vi "PipelineDuty.vi"(8 "error in (no error)":errorcluster, 10 "DataExchange":T1, 11 "GRMActor in":refnum<class "Displayer.lvclass">) -> (0 "error out":errorcluster, 2 "DataExchange  Out":T1, 3 "GRMActor out":refnum<class "Displayer.lvclass">)   [LabVIEW 2020, in "Displayer.lvlib" / "Displayer.lvclass"]
uses:
  Displayer.lvclass
  Model/Hardware Abstraction Layer/Component/Device/Device/DataExchange.ctl
  <vilib>/vision/Image Controls.llb/IMAQ Image.ctl
  Interface/DataListener Messages/OnDataChange Msg/OnDataChange Msg.lvclass/OnDataChange Msg.ctl
  <vilib>/ActorFramework/Message Enqueuer/Message Enqueuer.lvclass/Message Enqueuer.ctl
  <vilib>/ActorFramework/Message Enqueuer/Enqueue.vi
  Interface/DataListener Messages/OnDataChange Msg/OnDataChange Msg.lvclass
  C:/Program Files/National Instruments/LabVIEW 2020/vi.lib/ActorFramework/Message/Message.lvclass
  <vilib>/ActorFramework/Message Priority Queue/Priority Enqueue.vi
  Model/Hardware Abstraction Layer/Component/GenericActor/GenericActor/GenericActor.lvclass
  Interface/DataListener/DataListener.lvclass
panel:
  out "Source":string
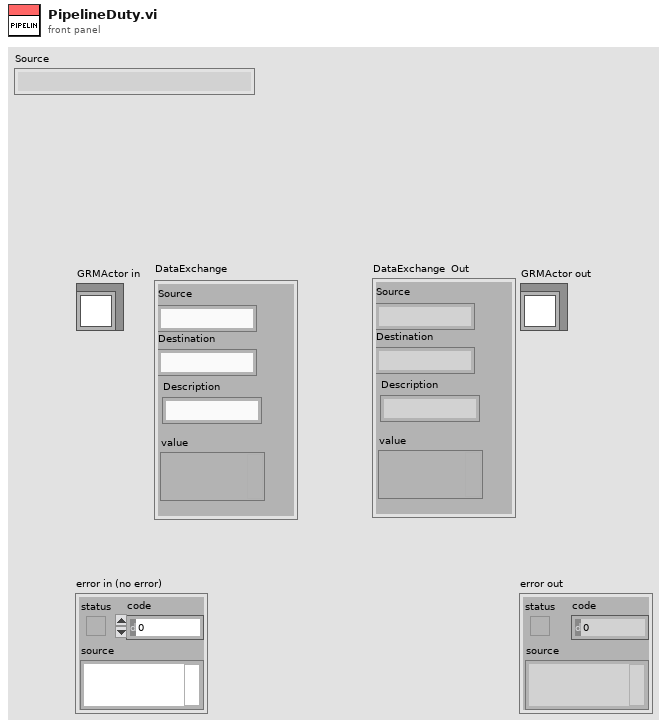
[diagram p1: front panel]
types:
  T1 = typedef "DataListener.lvclass/DataExchange.ctl" = cluster{"Source":string, "Destination":string, "Description":string, "value":variant}
  T2 = typedef "IMAQ Image.ctl" = refnum<image>
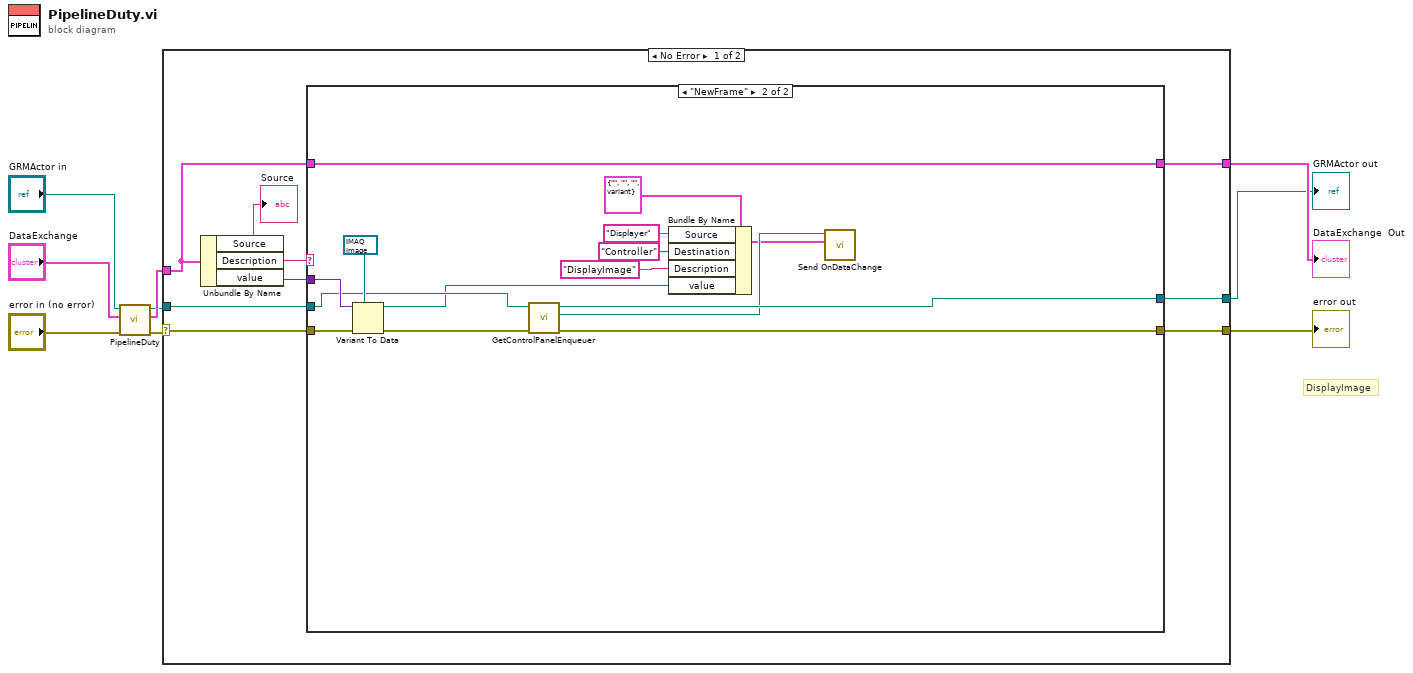
[diagram p0: block diagram]
diagram:
  # "DisplayImage"
  n1 = call-parent "PipelineDuty.vi"("error in (no error)"="error in (no error)", "DataExchange"="DataExchange", "GRMActor in"="GRMActor in") -> ("error out"=w6:errorcluster, "DataExchange 2"=w5:T1, "GRMActor out"=w4:refnum<class "Displayer.lvclass">)  [unwired: 6 in]
  n2 = case shown="No Error" w6 {
    selector: w6 -> [w16 w39]
    tunnel: [w17 w39] -> w2
    tunnel: w4 -> [w13 w38]
    tunnel: [w18 w38] -> w1
    tunnel: w5 -> [w12 w37]
    tunnel: [w11 w37] -> w3
    frame No Error {
      n3 = Unbundle By Name(w12) -> ("Source"=→"Source":string, "Description"=w15:string, "value"=w14:variant)
      n4 = case shown="\"NewFrame\"" w15 {
        tunnel: w14 -> [_ w35]
        tunnel: [w21 w29] -> w18
        tunnel: w13 -> [w21 w30]
        tunnel: [w20 w31] -> w17
        tunnel: w16 -> [w20 w36]
        tunnel: w12 -> [w19 w32]
        tunnel: [w19 w32] -> w11
        frame Default {
        }
        frame "NewFrame" {
          n5 = Variant To Data(error in=w36, type=T2 refnum ("New Image"), Variant=w35) -> (data=w22:T2, error out=w33:errorcluster)
          n6 = call-dynamic "GetControlPanelEnqueuer.vi"("error in (no error)"=w33, "GRMActor in"=w30) -> ("error out"=w31:errorcluster, "ControlViewEnqueuer"=w28:refnum<class "Message Enqueuer.lvclass">, "GRMActor out"=w29:refnum<class "Displayer.lvclass">)  [unwired: 7 in]
          n7 = Bundle By Name(cluster=T1 {"Source"="", "Destination"="", "Description"="", "value"=variant} ("DataExchange"), "Source"="Displayer", "Destination"="Controller", "Description"="DisplayImage", "value"=w22) -> (w26:T1)
          n8 = call "Send OnDataChange.vi"("DataExchange"=w26, "Message Enqueuer"=w28) -> ()  [unwired: 8 in, 2 out]
        }
      }
    }
    frame Error {
    }
  }
  "error out" <- w2
  "GRMActor out" <- w1
  "DataExchange  Out" <- w3
